vi "AlgorithmASolenoidAngleandPosition.vi"(2 "Theta in degrees":dbl, 3 "MartchBall Y":dbl) -> (0 "Ymovement":dbl, 1 "X movefromcenter":dbl)   [LabVIEW 2014]
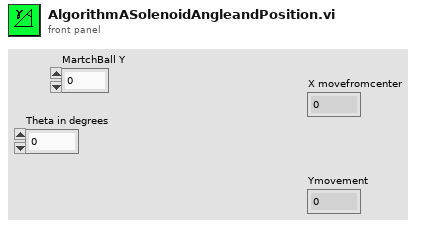
[diagram p1: front panel]
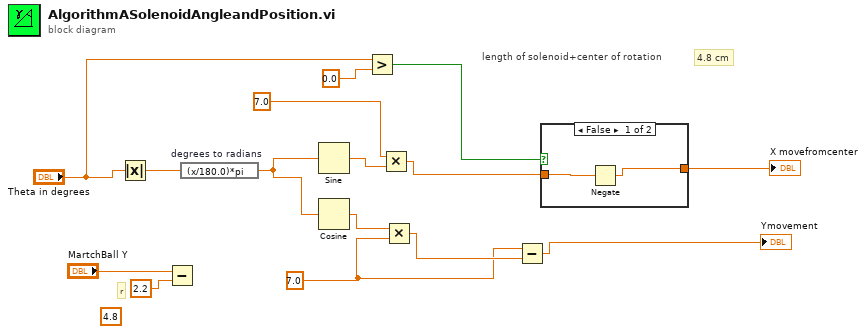
[diagram p0: block diagram]
diagram:
  w2 = 7.0
  (unwired) 4.8
  # "r"
  # "4.8 cm"
  # "length of solenoid+center of rotation"
  n1 = Absolute Value(x="Theta in degrees") -> (abs(x)=w14:dbl)
  n2 = Subtract(x="MartchBall Y", y=2.2) -> ()  [unwired: 1 out]
  n3 = expression code="(x/180.0)*pi" "degrees to radians"(w14) -> (w15:dbl)
  n4 = Sine(x=w15) -> (sin(x)=w12:dbl)
  n5 = Cosine(x=w15) -> (cos(x)=w13:dbl)
  n6 = Greater?(x="Theta in degrees", y=0.0) -> (0:w11:bool)
  n7 = Multiply(x=7.0, y=w12) -> (x*y=w8:dbl)
  n8 = Multiply(x=w13, y=w2) -> (x*y=w6:dbl)
  n9 = Subtract(x=w2, y=w6) -> (x-y=→"Ymovement":dbl)
  n10 = case shown="False" w11 {
    tunnel: w8 -> [w16 w18]
    tunnel: [w17 w18] -> w7
    frame False {
      n11 = Negate(x=w16) -> (-x=w17:dbl)
    }
    frame True {
    }
  }
  "X movefromcenter" <- w7
